vi "Get Custom Fields.vi"(6 "Authentication Header":T2[](array[typedef]), 8 "error in (no error)":errorcluster, 10 "Workspace GID":string) -> (0 "error out":errorcluster, 3 "data":T1)   [LabVIEW 2016]
uses:
  <vilib>/addons/_JKI.lib/REST Client/classes/REST Client/HTTP Header.ctl
  <vilib>/addons/_JKI.lib/REST Client/classes/REST Client/REST Client.lvclass
  <vilib>/addons/_JKI.lib/Serialization/JSON/JKI JSON Serialization.lvlib
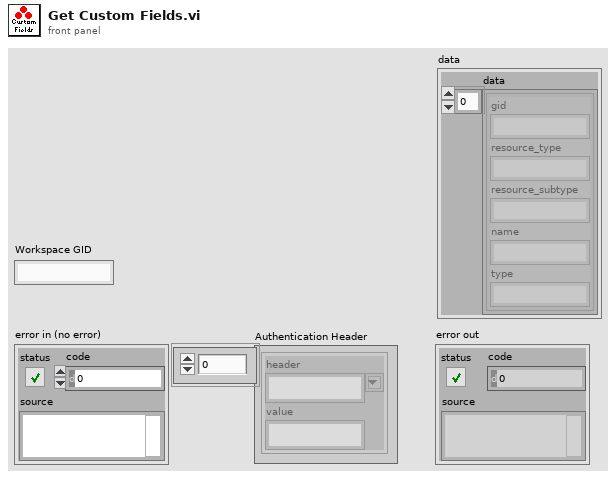
[diagram p1: front panel]
types:
  T1 = cluster{"data":cluster{"gid":string, "resource_type":string, "resource_subtype":string, "name":string, "type":string}[]}
  T2 = typedef "REST Client.lvlib/REST Client.lvclass/HTTP Header.ctl" = cluster{"header":string, "value":string}
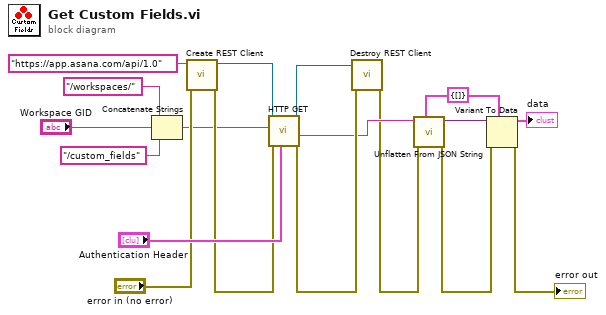
[diagram p0: block diagram]
diagram:
  w3 = T1 {"data"=[]}
  n1 = Concatenate Strings("/workspaces/", "Workspace GID", "/custom_fields") -> (w9:string)
  n2 = call <vilib>:"Create REST Client.vi"("error in (no error)"="error in (no error)", "Base URL"="https://app.asana.com/api/1.0") -> ("error out"=w14:errorcluster, "REST Client out"=w18:refnum<class "REST Client.lvclass">)  [unwired: 8 in]
  n3 = call-dynamic "HTTP GET.vi"("request specific headers"="Authentication Header", "error in (no error)"=w14, "Path"=w9, "REST Client in"=w18) -> ("error out"=w13:errorcluster, "Response body"=w8:string, "REST Client out"=w17:refnum<class "REST Client.lvclass">)  [unwired: 2 in, 3 out]
  n4 = call-dynamic "Destroy REST Client.vi"("error in (no error)"=w13, "REST Client in"=w17) -> ("error out"=w6:errorcluster)  [unwired: 9 in]
  n5 = call <vilib>:"Unflatten From JSON String.vi"("Type and Defaults"=w3, "error in (no error)"=w6, "JSON String"=w8) -> ("error out"=w4:errorcluster, "Variant"=w7:variant)  [unwired: 7 in]
  n6 = Variant To Data(error in=w4, type=w3, Variant=w7) -> (data=→"data":T1, error out=→"error out":errorcluster)
